vi "runScript.vi"(6 "timeStamp":string, 8 "error in (no error)":errorcluster, 9 "Path":path, 10 "CompiledScript":T1, 11 "HWController in":refnum<class "HWController.lvclass">) -> (0 "error out":errorcluster, 3 "HWController out":refnum<class "HWController.lvclass">)   [LabVIEW 2009, in "Hardware.lvlib" / "HWControllers.lvlib" / "HWController.lvclass"]
uses:
  HWController.lvclass
  Tools/SettingsProcessors/ScriptListCompiler/ScriptListCompiler.lvclass
  Channels/VoltOutput/AnalogOutput.lvclass
  Channels/Digital/DigitalOutput.lvclass
  Channels/DDSOutput/Generic/DDSOutput.lvclass
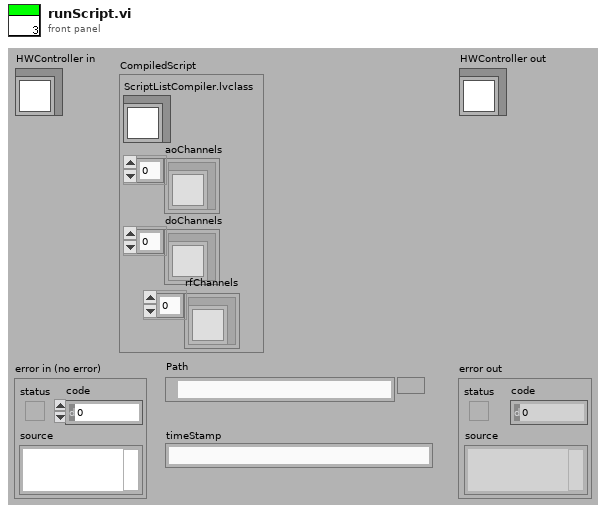
[diagram p1: front panel]
types:
  T1 = cluster{"ScriptListCompiler.lvclass":refnum<class "ScriptListCompiler.lvclass">, "aoChannels":refnum<class "AnalogOutput.lvclass">[], "doChannels":refnum<class "DigitalOutput.lvclass">[], "rfChannels":refnum<class "DDSOutput.lvclass">[]}
  T2 = enum16{"Ready", "Compiling", "Configured", "Running", "Stopping", "Unresolved Error"}
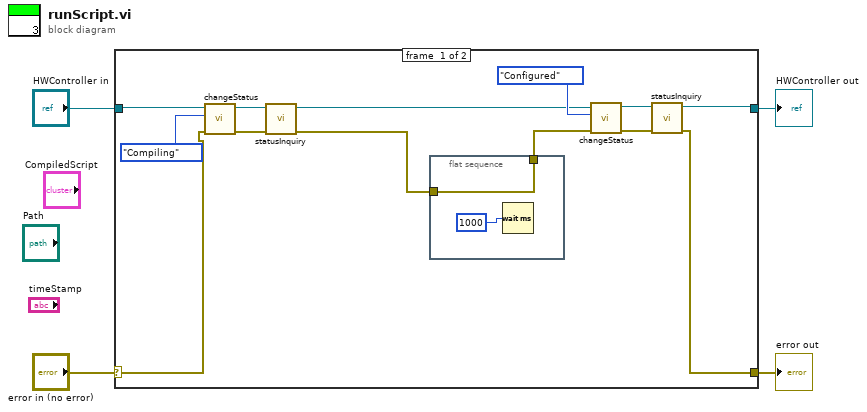
[diagram p0: block diagram]
diagram:
  n1 = case shown="No Error" "error in (no error)" {
    selector: "error in (no error)" -> [w9 w21]
    tunnel: [w6 w21] -> w3
    tunnel: [w11 w20] -> w1
    tunnel: "HWController in" -> [w10 w20]
    frame #0 {
      n2 = call "changeStatus.vi"("error in (no error)"=w9, "status"=T2."Compiling", "HWController in"=w10) -> ("error out"=w14:errorcluster, "HWController out"=w13:refnum<class "HWController.lvclass">)  [unwired: 7 in]
      n3 = call-dynamic "statusInquiry.vi"("error in (no error)"=w14, "HWController in"=w13) -> ("error out"=w5:errorcluster, "HWController out"=w8:refnum<class "HWController.lvclass">)  [unwired: 8 in]
      n4 = flat-sequence {
        tunnel: w5 -> [w18]
        tunnel: [w18] -> w7
        frame #0 {
          n5 = Wait (ms)(milliseconds to wait=1000) -> ()  [unwired: 1 out]
        }
      }
      n6 = call "changeStatus.vi"("error in (no error)"=w7, "status"=T2."Configured", "HWController in"=w8) -> ("error out"=w17:errorcluster, "HWController out"=w16:refnum<class "HWController.lvclass">)  [unwired: 7 in]
      n7 = call-dynamic "statusInquiry.vi"("error in (no error)"=w17, "HWController in"=w16) -> ("error out"=w6:errorcluster, "HWController out"=w11:refnum<class "HWController.lvclass">)  [unwired: 8 in]
    }
    frame #1 {
    }
  }
  "error out" <- w3
  "HWController out" <- w1
